vi "Write Power.vi"(8 "error in (no error)":errorcluster, 10 "Power":u8 caption="Power [8bit]", 11 "LaserPower in":refnum<class "LaserPower.lvclass">) -> (0 "error out":errorcluster, 3 "LaserPower out":refnum<class "LaserPower.lvclass">)   [LabVIEW 2013, in "HardwareCharacterization.lvlib" / "LaserPower.lvclass"]
uses:
  LaserPower.lvclass
  LaserPower.lvclass/LaserPower.ctl
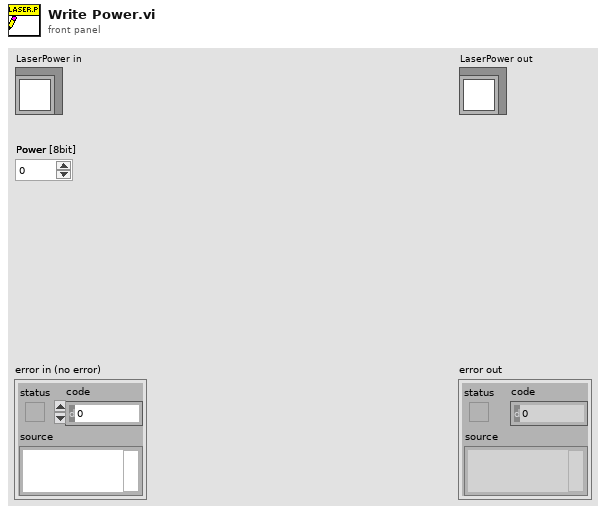
[diagram p1: front panel]
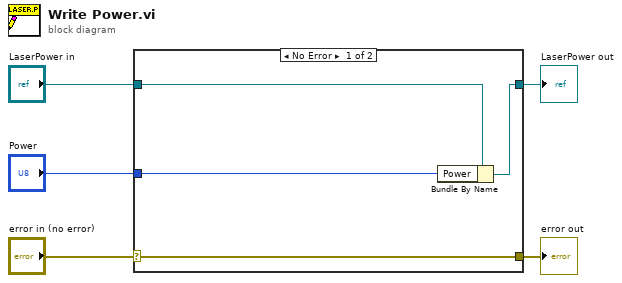
[diagram p0: block diagram]
diagram:
  n1 = case shown="No Error" "error in (no error)" {
    selector: "error in (no error)" -> [w9 w10]
    tunnel: [w9 w10] -> w4
    tunnel: [w7 w11] -> w2
    tunnel: "LaserPower in" -> [w8 w11]
    tunnel: "Power" -> [w6 _]
    frame No Error {
      n2 = Bundle By Name(cluster=w8, "Power"=w6) -> (w7:refnum<class "LaserPower.lvclass">)
    }
    frame Error {
    }
  }
  "error out" <- w4
  "LaserPower out" <- w2
